vi "nth Derivative of Rat Poly for PFE (CDB).vi"(9 "order":i32, 10 "Q(x)":cdb[](array[numeric]) format="%#.2g", 11 "P(x)":cdb[](array[numeric]) format="%#.2g") -> (0 "error":i32, 2 "Denominator d[P(x)/Q(x)]/dx":cdb[](array[numeric]) format="%#.2g", 3 "Numerator d[P(x)/Q(x)]/dx":cdb[](array[numeric]) format="%#.2g")   [LabVIEW 2017, in "NI_AALPro.lvlib"]
uses:
  <vilib>/Analysis/NI_AALPro.lvlib
  <vilib>/Analysis/polynomials.llb/Remove Zero Coefficients (CDB).vi
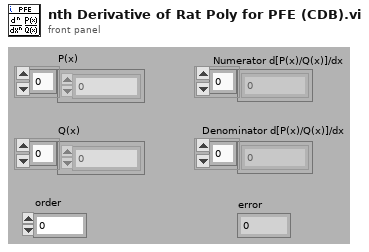
[diagram p1: front panel]
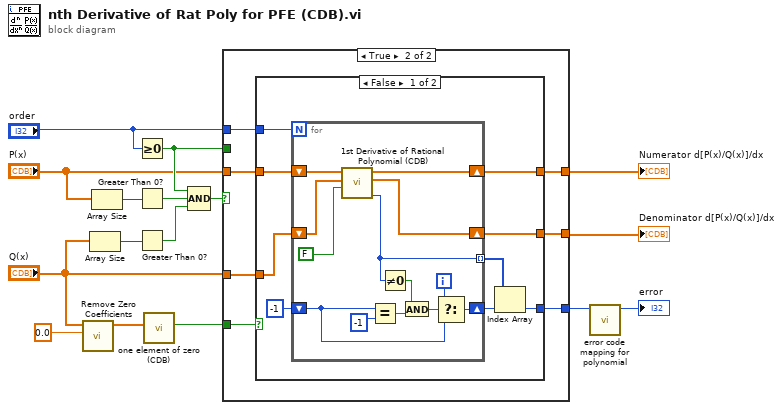
[diagram p0: block diagram]
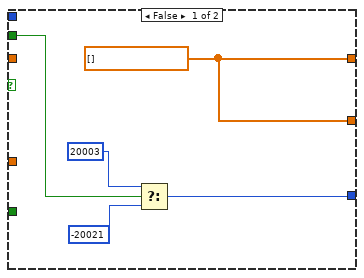
[diagram p2: hidden frame]
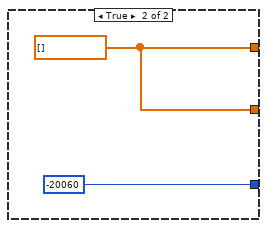
[diagram p3: hidden frame]
diagram:
  n1 = call-poly <vilib>:"Remove Zero Coefficients.vi"("threshold"=0.0, "P(x) In"="Q(x)") -> ("P(x) Out"=w7:cdb[])  [unwired: 7 in, 2 out]
  n2 = Array Size(array="Q(x)") -> (size(s)=w8:i32)
  n3 = Array Size(array="P(x)") -> (size(s)=w9:i32)
  n4 = Greater Or Equal To 0?(x="order") -> (x >= 0?=w5:bool)
  n5 = Greater Than 0?(x=w9) -> (x > 0?=w12:bool)
  n6 = Greater Than 0?(x=w8) -> (x > 0?=w11:bool)
  n7 = call <vilib>:"one element of zero (CDB).vi"("Array in"=w7) -> ("equal [0]?"=w6:bool)  [unwired: 10 in]
  n8 = Compound Arithmetic op=AND(w5, w12, w11) -> (w10:bool)
  n9 = case shown="True" w10 {
    tunnel: "P(x)" -> [_ w28]
    tunnel: "order" -> [_ w24]
    tunnel: [w21 w27] -> w16
    tunnel: "Q(x)" -> [_ w26]
    tunnel: [w21 w25] -> w15
    tunnel: w6 -> [_ w23]
    tunnel: w5 -> [w20 _]
    tunnel: [w17 w22] -> w4
    frame False {
      w21 = cdb[] [] ("Numerator d[p(s)/q(s)]/ds")
      n10 = Select(t=20003 ("empty array"), s=w20, f=-20021 ("minus order")) -> (s? t:f=w17:i32)
    }
    frame True {
      n11 = case shown="False" w23 {
        tunnel: w28 -> [w37 _]
        tunnel: [w36 w52] -> w27
        tunnel: w26 -> [w35 _]
        tunnel: [w34 w52] -> w25
        tunnel: w24 -> [w33 _]
        tunnel: [w29 -20060 ("divide by zero")] -> w22
        frame False {
          n12 = for {
            N: w33 -> [_]
            shift-right: [w41] -> w36
            shift-left: w37 -> [w43]
            shift-right: [w40] -> w34
            shift-left: w35 -> [w42]
            shift-right: [w44] -> w31
            shift-left: -1 -> [w45]
            tunnel: [w39] -> w30 mode=indexing
            i -> [w46]
            n13 = call <vilib>:"1st Derivative of Rational Polynomial (CDB).vi"("GCD?"=FALSE, "Q(x)"=w42, "P(x)"=w43) -> ("error"=w39:i32, "Denominator d[P(x)/Q(x)]/dx"=w40:cdb[], "Numerator d[P(x)/Q(x)]/dx"=w41:cdb[])  [unwired: 6 in]
            n14 = Equal?(x=w45, y=-1) -> (x = y?=w49:bool)
            n15 = Not Equal To 0?(x=w39) -> (x != 0?=w48:bool)
            n16 = And(x=w48, y=w49) -> (x .and. y?=w47:bool)
            n17 = Select(t=w46, s=w47, f=w45) -> (s? t:f=w44:i32)
          }
          n18 = Index Array(array=w30, index=w31) -> (element=w29:i32)
        }
        frame True {
          w52 = cdb[] [] ("CDB")
        }
      }
    }
  }
  "Denominator d[P(x)/Q(x)]/dx" <- w15
  "Numerator d[P(x)/Q(x)]/dx" <- w16
  n19 = call <vilib>:"error code mapping for polynomial.vi"("error in"=w4) -> ("error out"=→"error":i32)  [unwired: 10 in]
